vi "MW区发.vi"(6 "数值类型":enum16{"长整型", "双精度"}(ring), 7 "MD模式":enum16{"读MD", "写MD"}(ring), 8 "值":sgl format="%.3g", 9 "值":i32=10, 10 "寄存器MD地址":i32=10, 11 "处理识别码":i32) -> (3 "String":string)   [LabVIEW 2016]
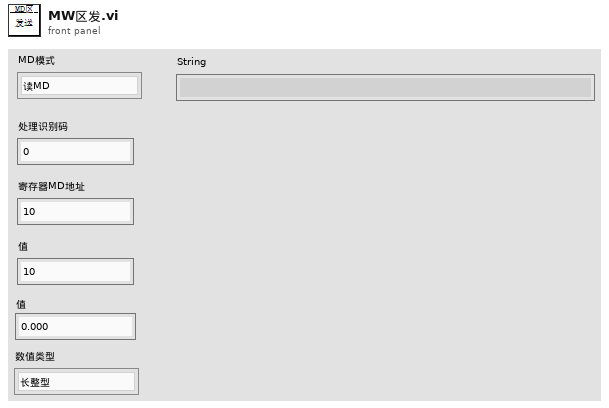
[diagram p1: front panel]
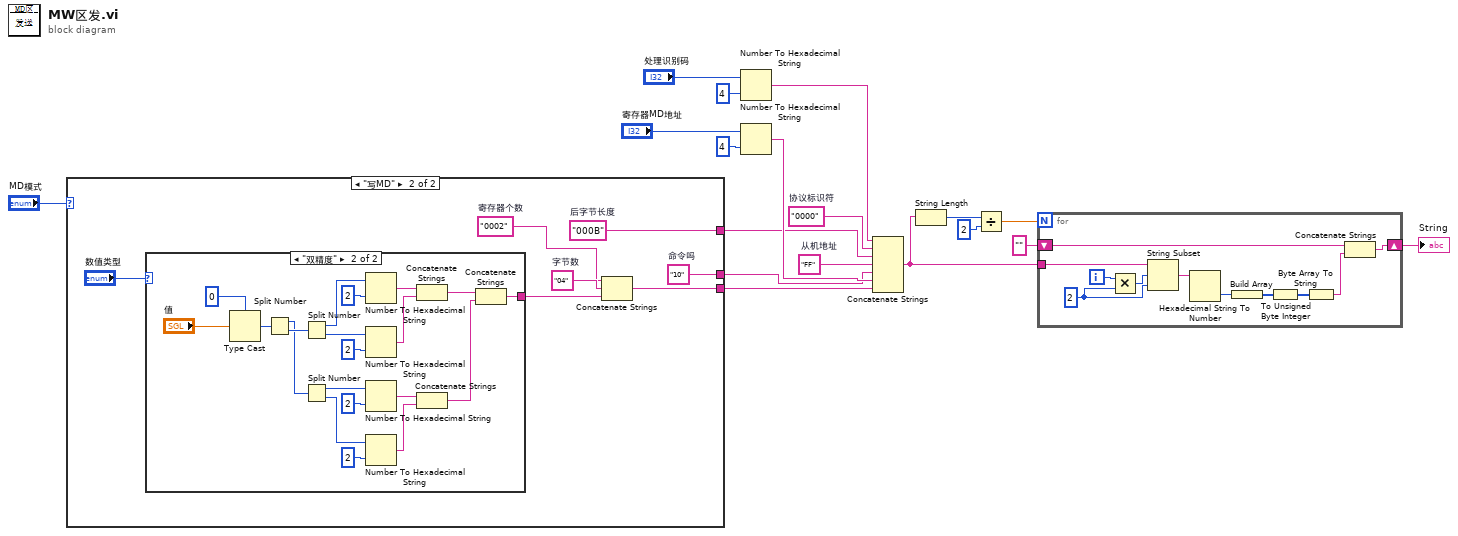
[diagram p0: block diagram]
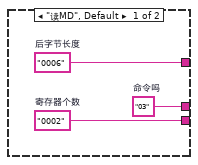
[diagram p2: hidden frame]
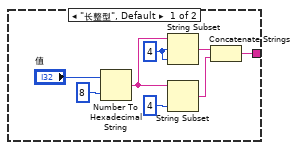
[diagram p3: hidden frame]
diagram:
  w13 = "FF"  # 从机地址
  w14 = "0000"  # 协议标识符
  n1 = case shown="\"写MD\"" "MD模式" {
    tunnel: [w21 w28] -> w4
    tunnel: [w20 w25] -> w3
    tunnel: [w19 w24] -> w2
    frame "读MD", Default {
      w19 = "03"  # 命令吗
      w20 = "0002"  # 寄存器个数
      w21 = "0006"  # 后字节长度
    }
    frame "写MD" {
      w24 = "10"  # 命令吗
      w27 = "04"  # 字节数
      w26 = "0002"  # 寄存器个数
      w28 = "000B"  # 后字节长度
      n2 = case shown="\"双精度\"" "数值类型" {
        tunnel: [w29 w37] -> w22
        frame "长整型", Default {
          w30 = 4 ("长度（剩余）")
          n3 = Number To Hexadecimal String(1:i16 8 ("宽度(-)"), 2:"值") -> (0:w31:string)
          n4 = String Subset(string=w31, offset (0)=w30, length (rest)=w30) -> (substring=w35:string)
          n5 = String Subset(string=w31, length (rest)=4 ("长度（剩余）")) -> (substring=w36:string)  [unwired: 1 in]
          n6 = Concatenate Strings(w35, w36) -> (w29:string)
        }
        frame "双精度" {
          n7 = Type Cast(type=0, x="值") -> (*(type *) &x=w40:i32)
          n8 = Split Number(x=w40) -> (hi(x)=w41:u16, lo(x)=w42:u16)
          n9 = Split Number(x=w42) -> (hi(x)=w49:u8, lo(x)=w50:u8)
          n10 = Split Number(x=w41) -> (hi(x)=w44:u8, lo(x)=w48:u8)
          n11 = Number To Hexadecimal String(1:i16 2 ("宽度(-)"), 2:w49) -> (0:w51:string)
          n12 = Number To Hexadecimal String(1:i16 2 ("宽度(-)"), 2:w50) -> (0:w52:string)
          n13 = Number To Hexadecimal String(1:i16 2 ("宽度(-)"), 2:w44) -> (0:w53:string)
          n14 = Number To Hexadecimal String(1:i16 2 ("宽度(-)"), 2:w48) -> (0:w54:string)
          n15 = Concatenate Strings(w51, w52) -> (w55:string)
          n16 = Concatenate Strings(w53, w54) -> (w56:string)
          n17 = Concatenate Strings(w55, w56) -> (w37:string)
        }
      }
      n18 = Concatenate Strings(w26, w27, w22) -> (w25:string)
    }
  }
  n19 = Number To Hexadecimal String(1:i16 4 ("宽度(-)"), 2:"处理识别码") -> (0:w15:string)
  n20 = Number To Hexadecimal String(1:i16 4 ("宽度(-)"), 2:"寄存器MD地址") -> (0:w12:string)
  n21 = Concatenate Strings(w15, w14, w4, w13, w2, w12, w3) -> (w7:string)
  n22 = String Length(string=w7) -> (length=w10:i32)
  n23 = Divide(x=w10, y=2 ("length")) -> (x/y=w8:dbl)
  n24 = for {
    N: w8 -> [_]
    tunnel: w7 -> [w66]
    shift-right: [w62] -> w6
    shift-left: "" ("String") -> [w63]
    i -> [w61]
    w57 = 2 ("length (rest)")
    n25 = Multiply(x=w61, y=w57) -> (x*y=w60:i32)
    n26 = String Subset(string=w66, offset (0)=w60, length (rest)=w57) -> (substring=w65:string)
    n27 = Hexadecimal String To Number(string=w65) -> (number=w67:u32)  [unwired: 2 in, 1 out]
    n28 = Build Array(w67) -> (w59:u32[])
    n29 = To Unsigned Byte Integer(number=w59) -> (unsigned 8bit integer=w58:u8[])
    n30 = Byte Array To String(unsigned byte array=w58) -> (string=w64:string)
    n31 = Concatenate Strings(w63, w64) -> (w62:string)
  }
  "String" <- w6
